vi "TIO Stream Read.vi"(8 "error in (no error)":errorcluster, 11 "TC Connection":T2={"Type"=enum."Serial", "URL"="serial:///dev/cu.usbserial-00000", "TO"=500, "Addr"=0, "Port"=0, "TCP"=refnum, "UDP"=refnum, "Route"=""}) -> (0 "error out":errorcluster, 1 "Payload":string, 2 "Type":T1(ring)=enum."RPC Request", 3 "TC Connection":T2={"Type"=enum."Serial", "URL"="serial:///dev/cu.usbserial-00000", "TO"=500, "Addr"=0, "Port"=0, "TCP"=refnum, "UDP"=refnum, "Route"=""}, 4 "Route":string, 5 "Routing Matches":bool)   [LabVIEW 2010]
uses:
  <userlib>/TIO Library 2010/TIO Serial Checksum CRC32.vi
panel:
  out "Routing Size":u8
  out "Payload Length":u16
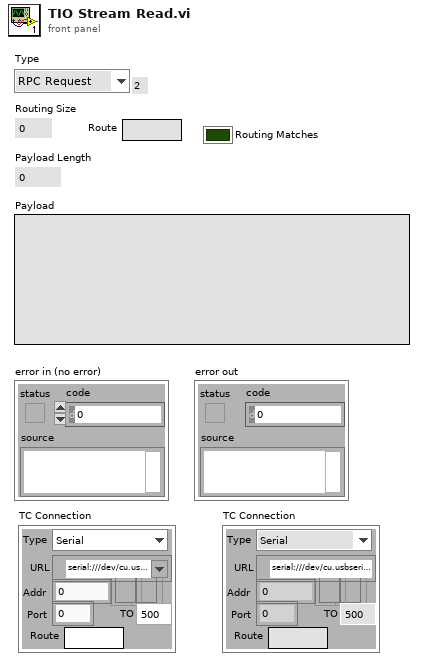
[diagram p1: front panel]
types:
  T1 = enum8{"Invalid", "Log", "RPC Request", "RPC Reply", "RPC Error", "Stream Description", "User"}
  T2 = cluster{"Type":enum16{"Serial", "TCP", "UDP", "mUDP"}, "URL":refnum<visa-resource-name>, "TO":u32, "Addr":u32, "Port":i32, "TCP":refnum<k5>, "UDP":refnum<k16>, "Route":string}
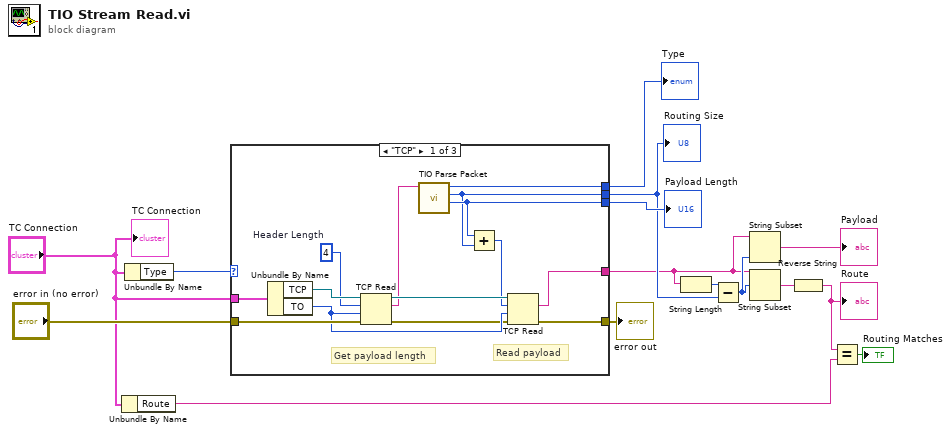
[diagram p0: block diagram]
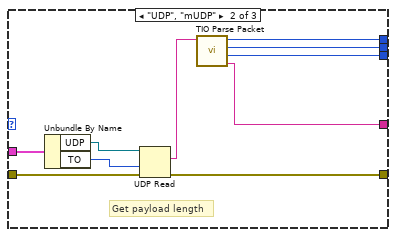
[diagram p2: hidden frame]
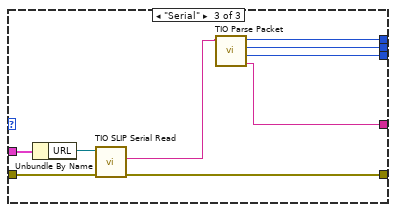
[diagram p3: hidden frame]
diagram:
  n1 = Unbundle By Name("TC Connection") -> ("Route"=w2:string)
  n2 = Unbundle By Name("TC Connection") -> ("Type"=w13:enum16{"Serial", "TCP", "UDP", "mUDP"})
  n3 = case shown="\"TCP\"" w13 {
    tunnel: "error in (no error)" -> [w26 w35 w47]
    tunnel: [w25 w30 w48] -> w15
    tunnel: "TC Connection" -> [w29 w39 w46]
    tunnel: [w24 w31 w41] -> w7
    tunnel: [w18 w37 w42] -> w12
    tunnel: [w17 w36 w43] -> w8
    tunnel: [w20 w38 w44] -> w11
    frame "TCP" {
      w22 = u32 4  # Header Length
      # "Read payload"
      # "Get payload length"
      n4 = Unbundle By Name(w29) -> ("TCP"=w28:refnum<k5>, "TO"=w23:u32)
      n5 = TCP Read(connection ID=w28, bytes to read=w22, error in (no error)=w26, 9:w23) -> (connection ID out=w27:refnum<k5>, data out=w21:string, error out=w19:errorcluster)  [unwired: 1 in]
      n6 = call <userlib>:"TIO Parse Packet.vi"("Packet"=w21) -> ("Payload Length"=w18:u16, "Routing Size"=w17:u8, "Type"=w20:u16)  [unwired: 7 in, 1 out]
      n7 = Add(x=w18, y=w17) -> (x+y=w16:u16)
      n8 = TCP Read(connection ID=w27, bytes to read=w16, error in (no error)=w19, 9:w23) -> (data out=w24:string, error out=w25:errorcluster)  [unwired: 1 in, 1 out]
    }
    frame "UDP", "mUDP" {
      # "Get payload length"
      n9 = Unbundle By Name(w39) -> ("UDP"=w34:refnum<k16>, "TO"=w33:u32)
      n10 = UDP Read(connection ID=w34, timeout ms (25000)=w33, 8:w35) -> (data out=w32:string, error out=w30:errorcluster)  [unwired: 1 in, 3 out]
      n11 = call <userlib>:"TIO Parse Packet.vi"("Packet"=w32) -> ("Payload"=w31:string, "Payload Length"=w37:u16, "Routing Size"=w36:u8, "Type"=w38:u16)  [unwired: 7 in]
    }
    frame "Serial" {
      n12 = Unbundle By Name(w46) -> ("URL"=w45:refnum<visa-resource-name>)
      n13 = call <userlib>:"TIO SLIP Serial Read.vi"("error in (no error)"=w47, "VISA resource name"=w45) -> ("error out"=w48:errorcluster, "Payload"=w40:string)  [unwired: 6 in, 2 out]
      n14 = call <userlib>:"TIO Parse Packet.vi"("Packet"=w40) -> ("Payload"=w41:string, "Payload Length"=w42:u16, "Routing Size"=w43:u8, "Type"=w44:u16)  [unwired: 7 in]
    }
  }
  "error out" <- w15
  "Type" <- w11
  "Routing Size" <- w8
  "Payload Length" <- w12
  n15 = String Length(string=w7) -> (length=w10:i32)
  n16 = Subtract(x=w10, y=w8) -> (x-y=w9:i32)
  n17 = String Subset(string=w7, length (rest)=w9) -> (substring=→"Payload":string)  [unwired: 1 in]
  n18 = String Subset(string=w7, offset (0)=w9) -> (substring=w4:string)  [unwired: 1 in]
  n19 = Reverse String(1:w4) -> (0:w1:string)
  "Route" <- w1
  n20 = Equal?(x=w1, y=w2) -> (x = y?=→"Routing Matches":bool)
  "TC Connection" <- "TC Connection"
